vi "Monedas Actualizadas.vi"(8 "error in (no error)":errorcluster, 10 "Monedas":cluster{"Numeric":dbl, "Boolean":bool}[](array[cluster])) -> (0 "error out":errorcluster)   [LabVIEW 2020]
doc: "Actualiza el valor de las monedas y si estan visibles o no\n_____\nCreated using Delacor QMH Event Scripter 5.0.0.112."
uses:
  Monedas Actualizadas Argument--cluster.ctl
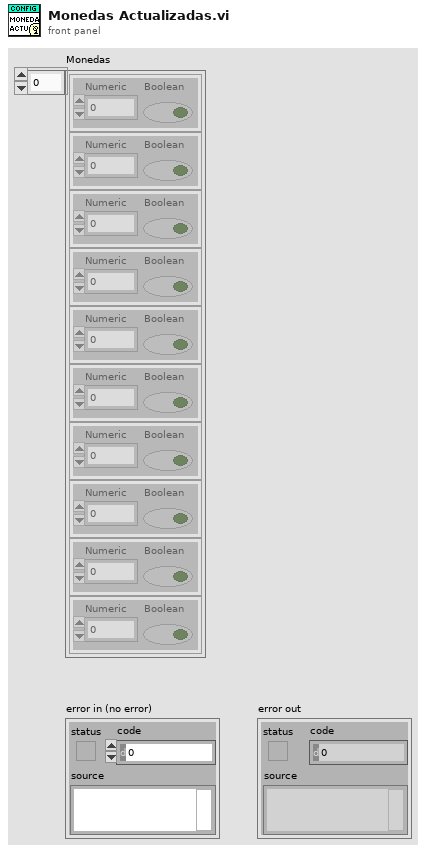
[diagram p1: front panel]
types:
  T1 = typedef "Monedas Actualizadas Argument--cluster.ctl" = cluster{"Monedas":cluster{"Numeric":dbl, "Boolean":bool}[]}
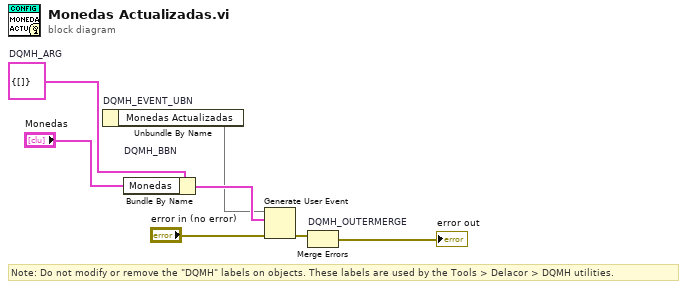
[diagram p0: block diagram]
diagram:
  w2 = T1 {"Monedas"=[]}  # DQMH_ARG
  # "Note: Do not modify or remove the \"DQMH\" labels on objects. These labels are used by the Tools > Delacor > DQMH utilities."
  n1 = Unbundle By Name "DQMH_EVENT_UBN"() -> ("Monedas Actualizadas"=w4)  [unwired: 1 in]
  n2 = Bundle By Name "DQMH_BBN"(cluster=w2, "Monedas"="Monedas") -> (w5:T1)
  n3 = Generate User Event(user event=w4, event data cluster=w5, error in="error in (no error)") -> (error out=w3:errorcluster)  [unwired: 1 in, 1 out]
  n4 = Merge Errors "DQMH_OUTERMERGE"(w3) -> (→"error out":errorcluster)  [unwired: 1 in]
